vi "sub Exit.vi"(8 "error in (no error)":errorcluster, 11 "LF2R IDE in":refnum<class "Main Panel.lvclass">) -> (0 "error out":errorcluster, 3 "LF2R IDE out":refnum<class "Main Panel.lvclass">)   [LabVIEW 2018, in "Main Panel.lvlib" / "Main Panel.lvclass"]
uses:
  Main Panel.lvclass
  C:/Program Files (x86)/National Instruments/LabVIEW 2018/vi.lib/ActorFramework/Actor/Actor.lvclass
  Main Panel.lvclass/Main Panel.ctl
  <vilib>/ActorFramework/Actor/Actor.lvclass/Actor.ctl
  <vilib>/ActorFramework/Message Enqueuer/Message Enqueuer.lvclass/Message Enqueuer.ctl
  <vilib>/ActorFramework/Message Enqueuer/Init from Existing Queue.vi
  <vilib>/ActorFramework/Message Enqueuer/Enqueue.vi
  <vilib>/ActorFramework/Stop Msg/Stop Msg.lvclass
  C:/Program Files (x86)/National Instruments/LabVIEW 2018/vi.lib/ActorFramework/Message/Message.lvclass
  <vilib>/ActorFramework/Message Priority Queue/Priority Enqueue.vi
  <vilib>/ActorFramework/Message Enqueuer/Message Enqueuer.lvclass
  <vilib>/ActorFramework/Actor/Actor.lvclass
  ScintillaNET/ScintillaNET.lvclass
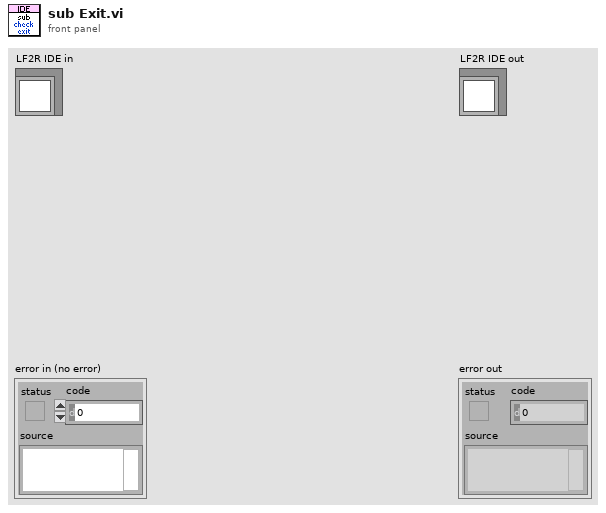
[diagram p1: front panel]
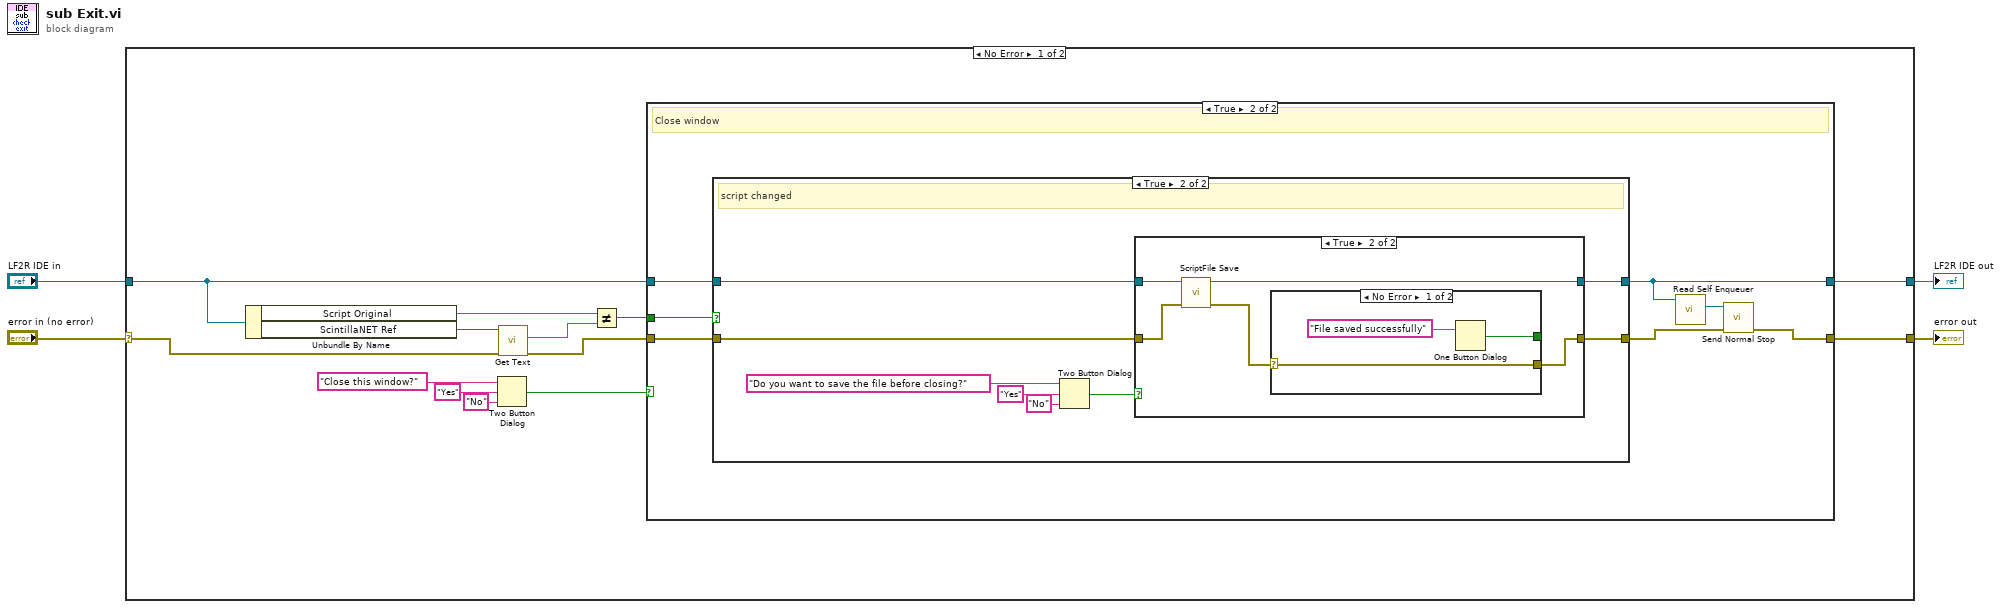
[diagram p0: block diagram]
diagram:
  n1 = case shown="No Error" "error in (no error)" {
    selector: "error in (no error)" -> [w6 w49]
    tunnel: [w10 w49] -> w3
    tunnel: [w11 w48] -> w1
    tunnel: "LF2R IDE in" -> [w12 w48]
    frame No Error {
      n2 = Unbundle By Name(w12) -> ("Script Original"=w14:string, "ScintillaNET Ref"=w9:refnum<class "ScintillaNET.lvclass">)
      n3 = Two Button Dialog(message="Close this window?", 1:"No" ("F button name (\"Cancel\")"), 2:"Yes" ("T button name (\"OK\")")) -> (T button?=w5:bool)
      n4 = call "Get Text.vi"("error in (no error)"=w6, "ScintillaNET in"=w9) -> ("error out"=w7:errorcluster, "Text"=w8:string)  [unwired: 7 in, 1 out]
      n5 = Not Equal?(x=w14, y=w8) -> (x != y?=w13:bool)
      n6 = case shown="True" w5 {
        tunnel: w13 -> [_ w26]
        tunnel: w12 -> [w19 w25]
        tunnel: [w19 w23] -> w11
        tunnel: [w18 w22] -> w10
        tunnel: w7 -> [w18 w21]
        frame False {
          # "Cancel"
        }
        frame True {
          # "Close window"
          n7 = case shown="True" w26 {
            tunnel: w25 -> [w28 w32]
            tunnel: w21 -> [w27 w31]
            tunnel: [w28 w30] -> w23
            tunnel: [w27 w29] -> w24
            frame False {
            }
            frame True {
              # "script changed"
              n8 = Two Button Dialog(message="Do you want to save the file before closing?", 1:"No" ("F button name (\"Cancel\")"), 2:"Yes" ("T button name (\"OK\")")) -> (T button?=w33:bool)
              n9 = case shown="True" w33 {
                tunnel: w32 -> [w37 w43]
                tunnel: w31 -> [w38 w42]
                tunnel: [w37 w41] -> w30
                tunnel: [w38 w39] -> w29
                frame False {
                }
                frame True {
                  n10 = call "ScriptFile Save.vi"("error in (no error)"=w42, "LF2R IDE in"=w43) -> ("error out"=w40:errorcluster, "LF2R IDE out"=w41:refnum<class "Main Panel.lvclass">)  [unwired: 7 in, 1 out]
                  n11 = case shown="No Error" w40 {
                    selector: w40 -> [w45 w47]
                    tunnel: [w45 w47] -> w39
                    tunnel: [w44 _] -> _
                    frame No Error {
                      n12 = One Button Dialog(message="File saved successfully") -> (true=w44:bool)  [unwired: 1 in]
                    }
                    frame Error {
                    }
                  }
                }
              }
            }
          }
          n13 = call <vilib>:"Read Self Enqueuer.vi"("Actor"=w23) -> ("Self Enqueuer"=w20:refnum<class "Message Enqueuer.lvclass">)  [unwired: 10 in]
          n14 = call <vilib>:"Send Normal Stop.vi"("error in (no error)"=w24, "Message Enqueuer"=w20) -> ("error out"=w22:errorcluster)  [unwired: 9 in]
        }
      }
    }
    frame Error {
    }
  }
  "error out" <- w3
  "LF2R IDE out" <- w1
